vi "exercices.vi"() -> ()   [LabVIEW 2020]
panel:
  out "area":dbl
  in  "base":dbl
  in  "height":dbl
  out "radian":dbl
  out "sine":dbl
  in  "degree":dbl
  out "felhenchtqin":dbl
  in  "celcus":dbl
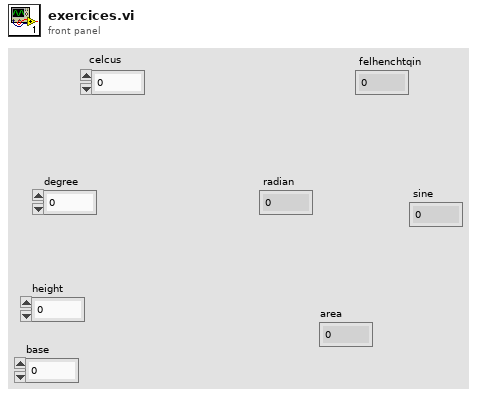
[diagram p1: front panel]
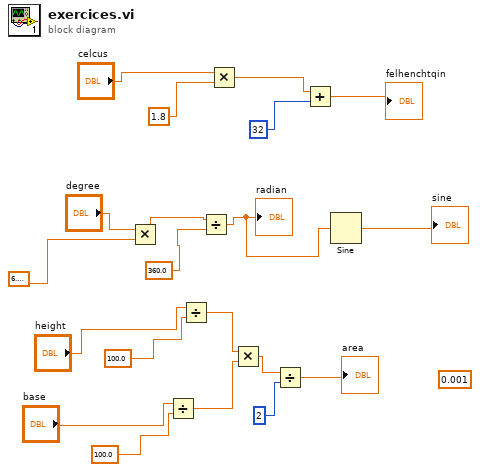
[diagram p0: block diagram]
diagram:
  (unwired) 0.001
  n1 = Multiply(x="degree", y=6.283185307179586) -> (x*y=w14:dbl)
  n2 = Divide(x="base", y=100.0) -> (x/y=w1:dbl)
  n3 = Divide(x="height", y=100.0) -> (x/y=w4:dbl)
  n4 = Divide(x=w14, y=360.0) -> (x/y=w12:dbl)
  "radian" <- w12
  n5 = Multiply(x="celcus", y=1.8) -> (x*y=w18:dbl)
  n6 = Multiply(x=w4, y=w1) -> (x*y=w9:dbl)
  n7 = Divide(x=w9, y=2) -> (x/y=→"area":dbl)
  n8 = Add(x=w18, y=32) -> (x+y=→"felhenchtqin":dbl)
  n9 = Sine(x=w12) -> (sin(x)=→"sine":dbl)
